vi "Read All Elements GUI.vi"(8 "error in (no error)":errorcluster, 11 "Mapping params in":refnum<class "CV-Mapping.lvclass">) -> (0 "error out":errorcluster, 2 "Mapping params.":T1={"Enable mapping"=FALSE, "Automatic timing"=FALSE, "Scan pattern file"=path "C:/CameraVision/Scan patterns/Template.sp", "Start off-set"=0.0, "Default map characteristic"=enum."Average intensity [0-255]", "Default mark speed"=1000, "Jump speed"=10000} {"Jump speed" min=1; "Default mark speed" min=1; "Start off-set" step=0.0001}, 3 "Mapping params out":refnum<class "CV-Mapping.lvclass">)   [LabVIEW 2013, in "CameraVision.lvlib" / "CV-Mapping.lvclass"]
uses:
  CV-Mapping.lvclass
  Mapping-parameters-gui.ctl
  Mapping-characteristic.ctl
  CV-Mapping.lvclass/CV-Mapping.ctl
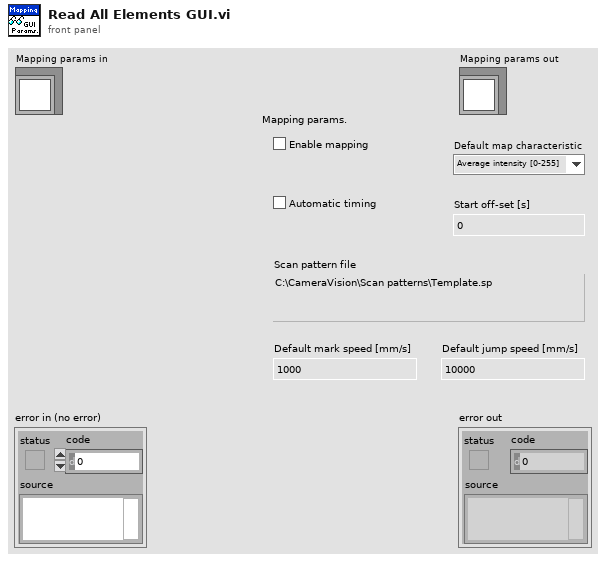
[diagram p1: front panel]
types:
  T1 = typedef "CameraVision.lvlib/CV-Mapping.lvclass/Mapping-parameters-gui.ctl" = cluster{"Enable mapping":bool, "Automatic timing":bool, "Scan pattern file":path, "Start off-set":dbl, "Default map characteristic":T2, "Default mark speed":i32, "Jump speed":i32}
  T2 = typedef "CameraVision.lvlib/CV-Mapping.lvclass/Mapping-characteristic.ctl" = enum16{"Average intensity [0-255]", "Peak intensity [0-255]", "Melt-pool size [mm²]", "Melt-pool aspect ratio []", "Melt-pool fragments []", "Average temperature [°C]", "Max. temperature [°C]", "Min. temperature [°C]", "Std. dev. temperature [°C]"}
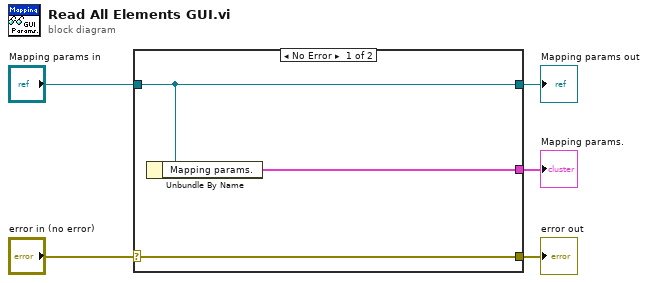
[diagram p0: block diagram]
diagram:
  n1 = case shown="No Error" "error in (no error)" {
    selector: "error in (no error)" -> [w8 w9]
    tunnel: [w8 w9] -> w4
    tunnel: [w7 w10] -> w2
    tunnel: "Mapping params in" -> [w7 w10]
    tunnel: [w6 _] -> w1
    frame No Error {
      n2 = Unbundle By Name(w7) -> ("Mapping params."=w6:T1)
    }
    frame Error {
    }
  }
  "error out" <- w4
  "Mapping params out" <- w2
  "Mapping params." <- w1
